vi "StartEqualization.vi"(8 "error in (no error)":errorcluster, 11 "reference in":refnum<class "sim_MmW.lvclass">) -> (0 "error out":errorcluster, 2 "channel":T1 {"frequency offset (Hz)" format="%#_6p"}, 3 "reference out":refnum<class "sim_MmW.lvclass">)   [LabVIEW 2019, in "sim_MmW.lvclass"]
doc: "Starts generating calibration pulse and prepares RX for acquisition"
uses:
  sim_MmW.lvclass
  C:/Barkhausen mmWave radar/Development/modules/mmw_instrument/src_LabVIEW/Host/SubVIs/mmWave instrument_class/mmWave instrument.lvclass
  mmWave instrument_class/Instrument state.ctl
  <vilib>/Utility/file.llb/Read Delimited Spreadsheet (string).vi
  mmWave instrument_class/mmWave instrument.lvclass
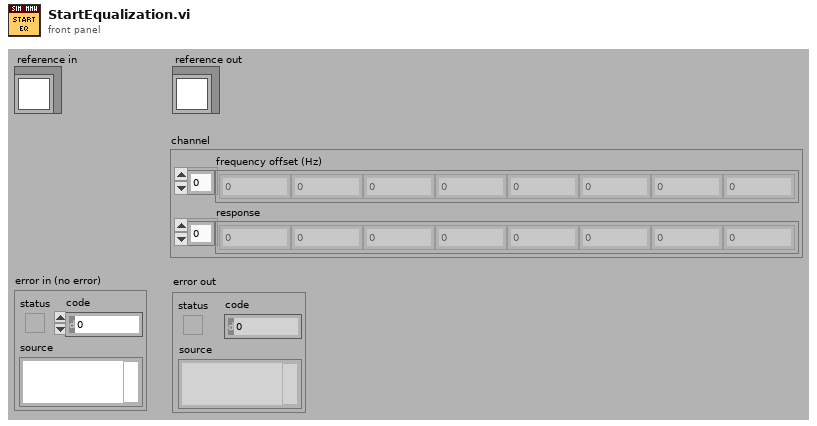
[diagram p1: front panel]
types:
  T1 = cluster{"frequency offset (Hz)":dbl[], "response":cdb[]}
  T2 = typedef "mmWave instrument.lvclass/Instrument state.ctl" = enum16{"Off", "Initialization", "Configuration", "Running", "Calibration"}
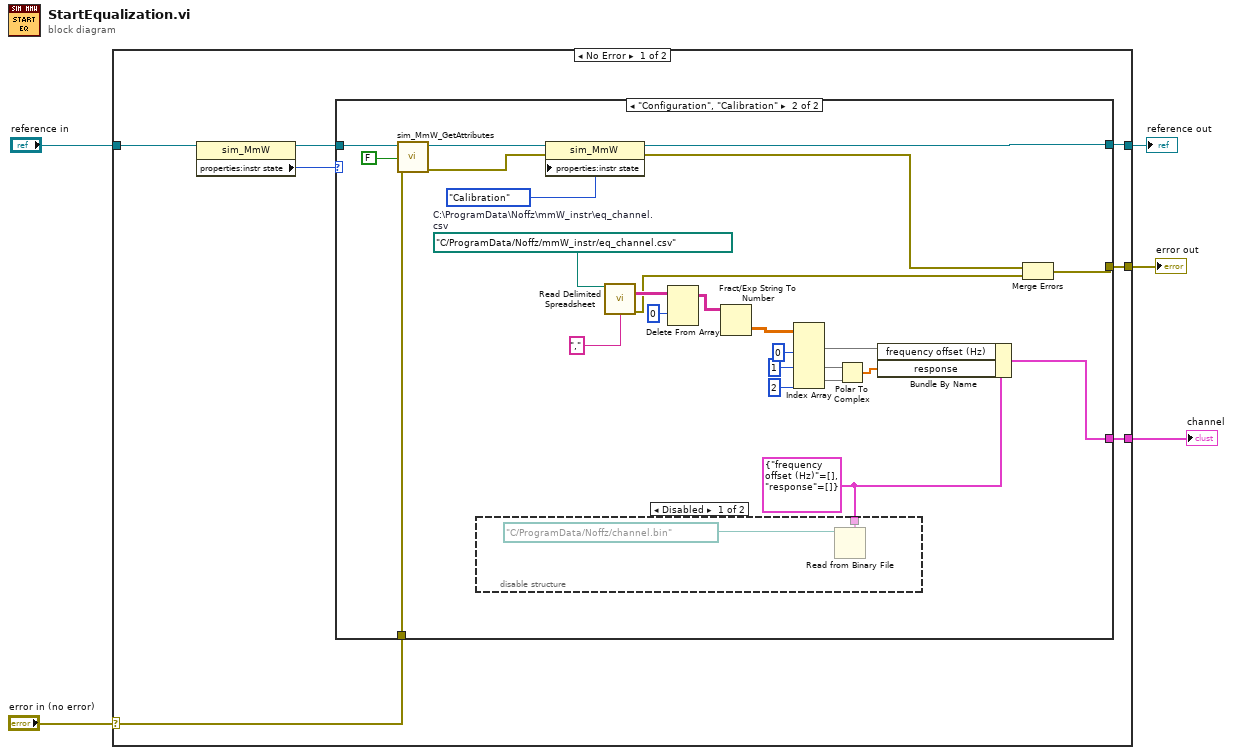
[diagram p0: block diagram]
diagram:
  n1 = case shown="No Error" "error in (no error)" {
    selector: "error in (no error)" -> [w12 w42]
    tunnel: [w7 w42] -> w4
    tunnel: [w9 w41] -> w2
    tunnel: "reference in" -> [w11 w41]
    tunnel: [w6 _] -> w1
    frame No Error {
      n2 = property class="sim_MmW"(reference=w11) -> (reference out=w10:refnum<class "sim_MmW.lvclass">, "properties:instr state"=w8:T2)  [unwired: 1 in, 1 out]
      n3 = case shown="\"Configuration\", \"Calibration\"" w8 {
        tunnel: w12 -> [_ w38]
        tunnel: w10 -> [w13 w36]
        tunnel: [w13 w34] -> w9
        tunnel: [_ w30] -> w7
        tunnel: [_ w19] -> w6
        frame "Off", Default {
        }
        frame "Configuration", "Calibration" {
          w29 = path "C:/ProgramData/Noffz/mmW_instr/eq_channel.csv"  # C:\ProgramData\Noffz\mmW_instr\eq_channel.csv
          w20 = T1 {"frequency offset (Hz)"=[], "response"=[]} ("channel")
          n4 = call "sim_MmW_GetAttributes.vi"("error in (no error)"=w38, "return data? (T)"=FALSE, "reference in"=w36) -> ("error out"=w32:errorcluster, "reference out"=w35:refnum<class "sim_MmW.lvclass">)  [unwired: 5 in, 2 out]
          n5 = disable-structure shown="Disabled" {
            disable-tunnel: w20 -> [w39 _]
            frame Disabled {
              n6 = Read from Binary File(5:w39, 11:path "C:/ProgramData/Noffz/channel.bin") -> ()  [unwired: 4 in, 4 out]
            }
            frame Enabled {
            }
          }
          n7 = property class="sim_MmW"(reference=w35, error in=w32, "properties:instr state"=Instrument_state."Calibration" ("instr state")) -> (reference out=w34:refnum<class "sim_MmW.lvclass">, error out=w31:errorcluster)
          n8 = call-poly <vilib>:"Read Delimited Spreadsheet.vi"("file path (dialog if empty)"=w29, "delimiter (\\t)"="," ("delimiter (\\t)")) -> ("all rows"=w27:string[][], "error out"=w14:errorcluster)  [unwired: 8 in, 4 out]
          n9 = Delete From Array(array=w27, index (row)=0) -> (array with subset deleted=w25:string[][])  [unwired: 2 in, 1 out]
          n10 = Fract/Exp String To Number(string=w25) -> (number=w24:dbl[][])  [unwired: 3 in, 1 out]
          n11 = Index Array(array=w24, index (col) #1=0 ("disabled index (col)"), index (col) #2=1 ("disabled index (col)"), index (col) #3=2 ("disabled index (col)")) -> (element #1=w18:dbl[], element #2=w17:dbl[], element #3=w16:dbl[])  [unwired: 3 in]
          n12 = Polar To Complex(1:w16, 2:w17) -> (0:w15:cdb[])
          n13 = Bundle By Name(cluster=w20, "frequency offset (Hz)"=w18, "response"=w15) -> (w19:T1)
          n14 = Merge Errors(w31, w14) -> (w30:errorcluster)
        }
      }
    }
    frame Error {
    }
  }
  "error out" <- w4
  "reference out" <- w2
  "channel" <- w1
